vi "setFlowRateSpec2.vi"(1 "Flow Rate (sccm)":dbl, 2 "Flow Range Index":u16(ring) items=["0-10 sccm", "0-100 sccm", "0-1000 sccm"], 3 "DA_Spec":T1) -> ()   [LabVIEW 2011]
uses:
  DA_Spec.ctl
  globals.vi
panel:
  # "Channel Index"
  # "Card Index"
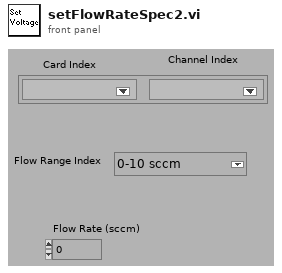
[diagram p1: front panel]
types:
  T1 = typedef "DA_Spec.ctl" = cluster{"Card Index":u16, "Channel Index":u16}
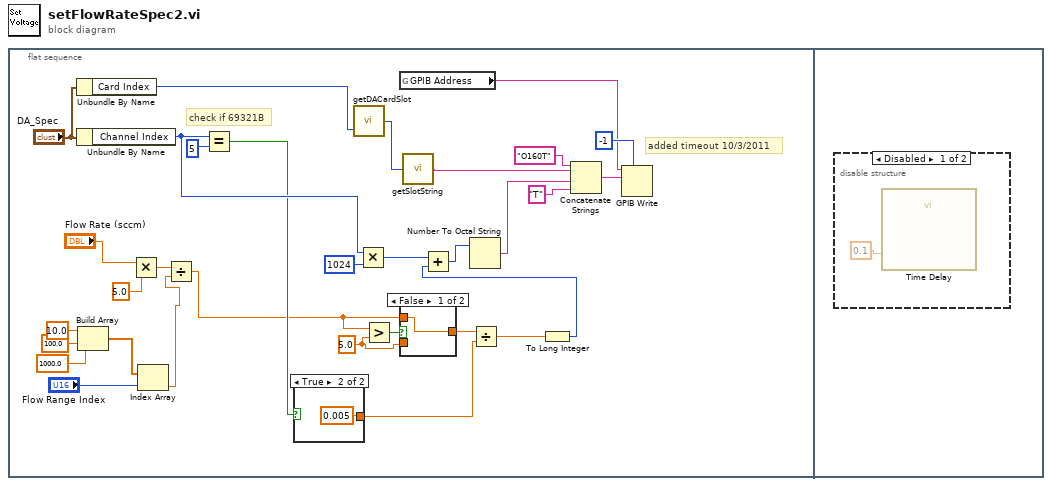
[diagram p0: block diagram]
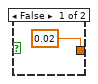
[diagram p3: hidden frame]
diagram:
  n1 = flat-sequence {
    frame #0 {
      w26 = 5.0 ("y")
      # "check if 69321B"
      # "added timeout 10/3/2011"
      n2 = Unbundle By Name("DA_Spec") -> ("Card Index"=w16:u16)
      n3 = Unbundle By Name("DA_Spec") -> ("Channel Index"=w13:u16)
      n4 = Build Array(10.0 ("element"), 100.0 ("element"), 1000.0 ("element")) -> (w4:dbl[])
      n5 = Multiply(x="Flow Rate (sccm)", y=5.0) -> (x*y=w10:dbl)
      n6 = Index Array(array=w4, index="Flow Range Index") -> (element=w3:dbl)
      n7 = Divide(x=w10, y=w3) -> (x/y=w2:dbl)
      n8 = Equal?(x=w13, y=u16 5) -> (x = y?=w11:bool)
      n9 = case shown="True" w11 {
        tunnel: [0.02 ("y") 0.005 ("y")] -> w20
        frame False {
        }
        frame True {
        }
      }
      n10 = call "getDACardSlot.vi"("Card Index"=w16) -> ("Slot"=w15:u16)  [unwired: 1 in]
      n11 = Multiply(x=w13, y=1024) -> (x*y=w31:i32)
      n12 = Greater?(x=w2, y=w26) -> (0:w25:bool)
      n13 = global read "globals.vi" "GPIB Address"() -> (w29:string)
      n14 = case shown="False" w25 {
        tunnel: w26 -> [_ w34]
        tunnel: [w33 w34] -> w27
        tunnel: w2 -> [w33 _]
        frame False {
        }
        frame True {
        }
      }
      n15 = call "getSlotString.vi"("Slot"=w15) -> ("string"=w17:string)
      n16 = Divide(x=w27, y=w20) -> (x/y=w30:dbl)
      n17 = To Long Integer(number=w30) -> (32bit integer=w21:i32)
      n18 = Add(x=w31, y=w21) -> (x+y=w23:i32)
      n19 = Number To Octal String(2:w23) -> (0:w24:string)  [unwired: 1 out]
      n20 = Concatenate Strings("O160T" ("string"), w17, w24, "T" ("string")) -> (w19:string)
      n21 = GPIB Write(0:w29, 1:w19, 4:-1 ("timeout ms (488.2 global)")) -> ()  [unwired: 1 in, 3 out]
    }
    frame #1 {
      n22 = disable-structure shown="Disabled" {
        frame Disabled {
          n23 = call "Time Delay"("Delay Time (s)"=0.1) -> ()  [unwired: 1 in, 10 out]
        }
        frame Enabled {
        }
      }
    }
  }
